vi "LogError.vi"(8 "error in (no error)":errorcluster, 10 "error":errorcluster, 11 "SimpleErrorLogger in":refnum<class "SimpleErrorLogger.lvclass">) -> (0 "error out":errorcluster, 3 "SimpleErrorLogger out":refnum<class "SimpleErrorLogger.lvclass">)   [LabVIEW 2023, in "SimpleErrorLogger.lvlib" / "SimpleErrorLogger.lvclass"]
uses:
  SimpleErrorLogger.lvclass
  SimpleErrorLogger.lvclass/SimpleErrorLogger.ctl
  <vilib>/ActorFramework/Actor/Actor.lvclass
  ApplicationWithErrorLogger Messages/FatalErrorOccurred Msg/FatalErrorOccurred Msg.lvclass
  SimpleErrorLogger Messages/Open Msg/Open Msg.lvclass
  <vilib>/ActorFramework/Stop Msg/Stop Msg.lvclass
  C:/Program Files (x86)/National Instruments/LabVIEW 2023/vi.lib/ActorFramework/Actor/Actor.lvclass
  C:/Source/LabVIEW/Error_Logger/SimpleErrorLogger/SimpleErrorLogger/SimpleErrorLogger.lvclass
  ApplicationWithErrorLogger Messages/ErrorCountUpdated Msg/ErrorCountUpdated Msg.lvclass
  SimpleErrorLogger Messages/LogError Msg/LogError Msg.lvclass
  <vilib>/ActorFramework/Message Enqueuer/Message Priority.ctl
  <vilib>/ActorFramework/Message Enqueuer/Message Enqueuer.lvclass
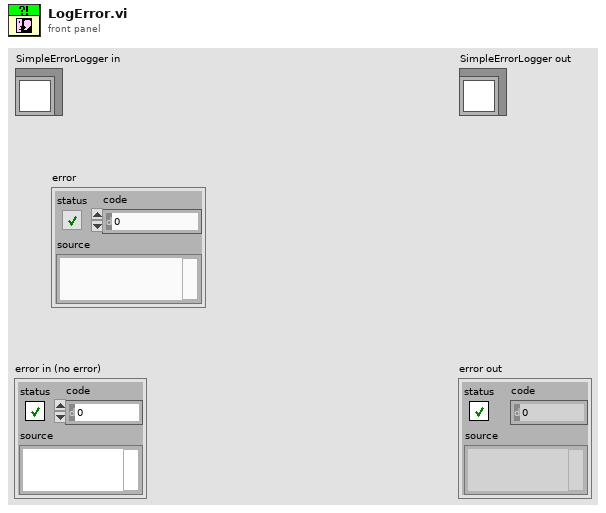
[diagram p1: front panel]
types:
  T1 = typedef "Actor Framework.lvlib/Message Enqueuer.lvclass/Message Priority.ctl" = enum16{"Low", "Normal", "High"}
  T2 = typedef "SimpleErrorLogger.lvlib/ErrorType.ctl" = enum16{"log", "fatal", "ignor"}
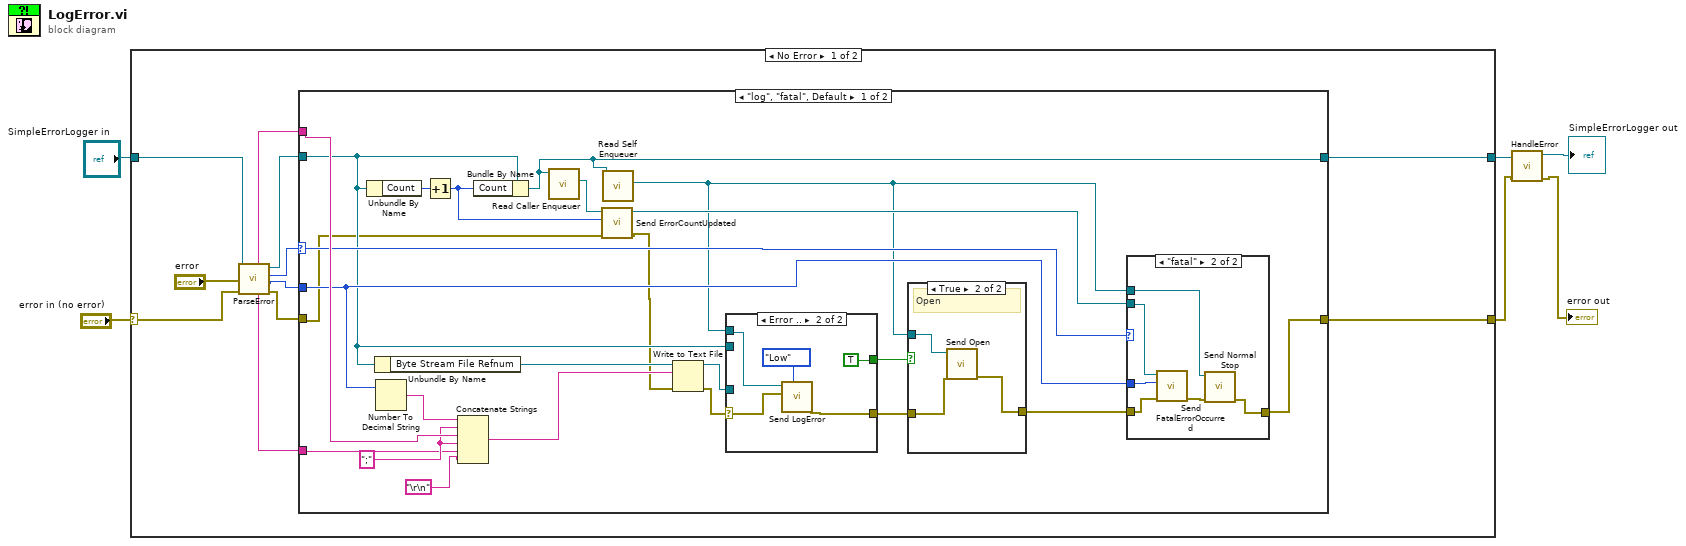
[diagram p0: block diagram]
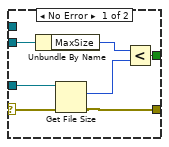
[diagram p4: hidden frame]
diagram:
  n1 = case shown="No Error" "error in (no error)" {
    selector: "error in (no error)" -> [w16 w68]
    tunnel: [w8 w68] -> w2
    tunnel: [w7 w67] -> w4
    tunnel: "SimpleErrorLogger in" -> [w17 w67]
    frame No Error {
      n2 = call "ParseError.vi"("error in (no error)"=w16, "error"="error", "SimpleErrorLogger in"=w17) -> ("error out"=w9:errorcluster, "Code"=w12:i32, "TypeOfError"=w13:T2, "SimpleErrorLogger out"=w14:refnum<class "SimpleErrorLogger.lvclass">, "Message"=w11:string, "source"=w10:string)  [unwired: 3 in]
      n3 = case shown="\"log\", \"fatal\", Default" w13 {
        selector: w13 -> [w30 _]
        tunnel: w14 -> [w25 w66]
        tunnel: w12 -> [w29 _]
        tunnel: w11 -> [w37 _]
        tunnel: w10 -> [w39 _]
        tunnel: w9 -> [w22 w65]
        tunnel: [w27 w65] -> w8
        tunnel: [w19 w66] -> w7
        frame "log", "fatal", Default {
          w38 = ";" ("string")
          n4 = Unbundle By Name(w25) -> ("Count"=w26:u32)
          n5 = Unbundle By Name(w25) -> ("Byte Stream File Refnum"=w41:refnum<file>)
          n6 = Number To Decimal String(number=w29) -> (decimal integer string=w40:string)  [unwired: 1 in]
          n7 = Increment(x=w26) -> (x+1=w23:u32)
          n8 = Concatenate Strings(w40, w38, w39, w38, w37, "\r\n") -> (w35:string)
          n9 = Bundle By Name(cluster=w25, "Count"=w23) -> (w19:refnum<class "SimpleErrorLogger.lvclass">)
          n10 = call <vilib>:"Read Caller Enqueuer.vi"("Actor"=w19) -> ("Caller Enqueuer"=w24:refnum<class "Message Enqueuer.lvclass">)  [unwired: 10 in]
          n11 = call "Send ErrorCountUpdated.vi"("error in (no error)"=w22, "ErrorCount"=w23, "Message Enqueuer"=w24) -> ("error out"=w21:errorcluster, "Message Enqueuer out"=w20:refnum<class "Message Enqueuer.lvclass">)  [unwired: 7 in]
          n12 = call <vilib>:"Read Self Enqueuer.vi"("Actor"=w19) -> ("Self Enqueuer"=w18:refnum<class "Message Enqueuer.lvclass">)  [unwired: 10 in]
          n13 = Write to Text File(file (use dialog)=w41, text=w35, error in=w21) -> (refnum out=w33:refnum<file>, error out=w34:errorcluster)  [unwired: 1 in, 1 out]
          n14 = case shown="Error .." w34 {
            selector: w34 -> [w58 w62]
            tunnel: w33 -> [w59 _]
            tunnel: w25 -> [w57 _]
            tunnel: [w54 TRUE] -> w32
            tunnel: [w53 w61] -> w31
            tunnel: w18 -> [_ w63]
            frame No Error {
              n15 = Unbundle By Name(w57) -> ("MaxSize"=w56:i64)
              n16 = Get File Size(file=w59, error in=w58) -> (size (in bytes)=w55:i64, 0:w53:errorcluster)  [unwired: 1 out]
              n17 = Less?(x=w56, y=w55) -> (x < y?=w54:bool)
            }
            frame Error {
              n18 = call "Send LogError.vi"("Message Priority (Normal)"=Message_Priority."Low", "error"=w62, "Message Enqueuer"=w63) -> ("error out"=w61:errorcluster)  [unwired: 7 in, 1 out]
            }
          }
          n19 = case shown="True" w32 {
            tunnel: w31 -> [w49 w52]
            tunnel: [w49 w51] -> w28
            tunnel: w18 -> [_ w50]
            frame False {
            }
            frame True {
              # "Open"
              n20 = call "Send Open.vi"("error in (no error)"=w52, "Message Enqueuer"=w50) -> ("error out"=w51:errorcluster)  [unwired: 8 in, 1 out]
            }
          }
          n21 = case shown="\"fatal\"" w30 {
            tunnel: w29 -> [_ w48]
            tunnel: w28 -> [w42 w47]
            tunnel: [w42 w45] -> w27
            tunnel: w20 -> [_ w44]
            tunnel: w18 -> [_ w43]
            frame "log", Default {
            }
            frame "fatal" {
              n22 = call "Send FatalErrorOccurred.vi"("error in (no error)"=w47, "Code"=w48, "Message Enqueuer"=w44) -> ("error out"=w46:errorcluster)  [unwired: 7 in, 1 out]
              n23 = call <vilib>:"Send Normal Stop.vi"("error in (no error)"=w46, "Message Enqueuer"=w43) -> ("error out"=w45:errorcluster)  [unwired: 9 in]
            }
          }
        }
        frame "ignor" {
        }
      }
    }
    frame Error {
    }
  }
  n24 = call "HandleError.vi"("error in (no error)"=w2, "SimpleErrorLogger in"=w4) -> ("error out"=→"error out":errorcluster, "SimpleErrorLogger out"=→"SimpleErrorLogger out":refnum<class "SimpleErrorLogger.lvclass">)  [unwired: 8 in]
